vi "FGVVideoAccuracy.vi"(6 "Operation":enum16{"Read", "Write"}(ring)=enum."Write", 11 "VideoAccuracy":dbl format="%#_13g") -> (3 "VideoAccuracy":dbl format="%#_13g")   [LabVIEW 2024]
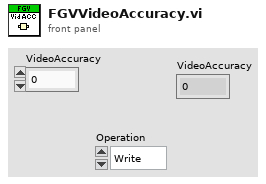
[diagram p1: front panel]
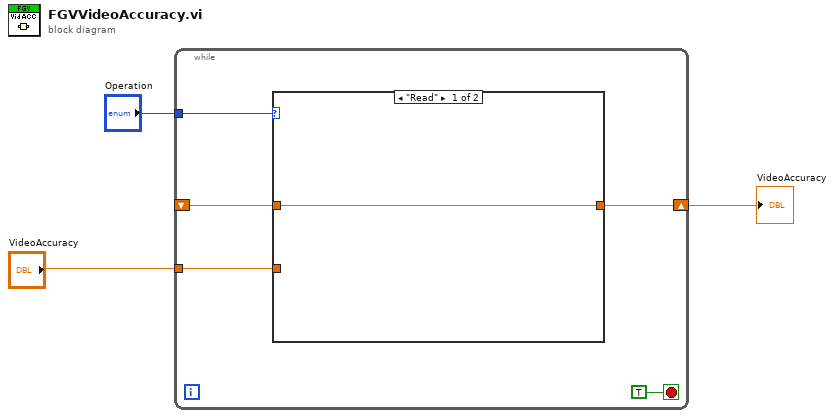
[diagram p0: block diagram]
diagram:
  n1 = while {
    tunnel: "VideoAccuracy" -> [w8]
    shift-right: [w7] -> w1
    shift-left: _ -> [w6]
    tunnel: "Operation" -> [w5]
    stop <- TRUE stop-if-true
    n2 = case shown="\"Read\"" w5 {
      tunnel: w8 -> [_ w10]
      tunnel: [w9 w10] -> w7
      tunnel: w6 -> [w9 _]
      frame "Read" {
      }
      frame "Write" {
      }
    }
  }
  "VideoAccuracy" <- w1
